vi "批次管理.vi"() -> ()   [LabVIEW 2020]
uses:
  <vilib>/addons/database/Connection.llb/DB Tools Open Connec (String).vi
  <vilib>/addons/database/Connection.llb/Conn Execute.vi
  <vilib>/addons/database/Recordset.llb/Rec Fetch Recordset Data (R).vi
  <vilib>/addons/database/Recordset.llb/Rec Destroy - Connection.vi
  Global_Variable/Global.vi
  <vilib>/addons/database/NI_Database_API.lvlib
panel:
  out "产品型号":string
  out "批次信息":string[][](table)
  # "批次管理"
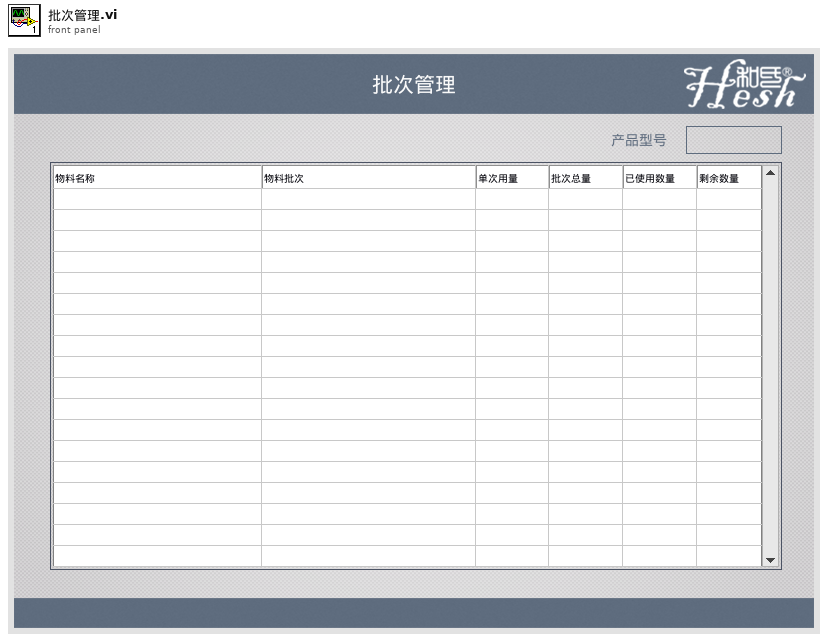
[diagram p1: front panel]
types:
  T1 = typedef "NI_Database_API.lvlib/Conn ObjectReference.ctl" = refnum<k1>
  T2 = typedef "NI_Database_API.lvlib/Rec ObjectReference.ctl" = refnum<k1>
  T3 = typedef "LVPoint32TypeDef.ctl" = cluster{"Horizontal":i32, "Vertical":i32}
  T4 = typedef "LVRowAndColumnTypeDef.ctl" = cluster{"Row":i32, "Column":i32}
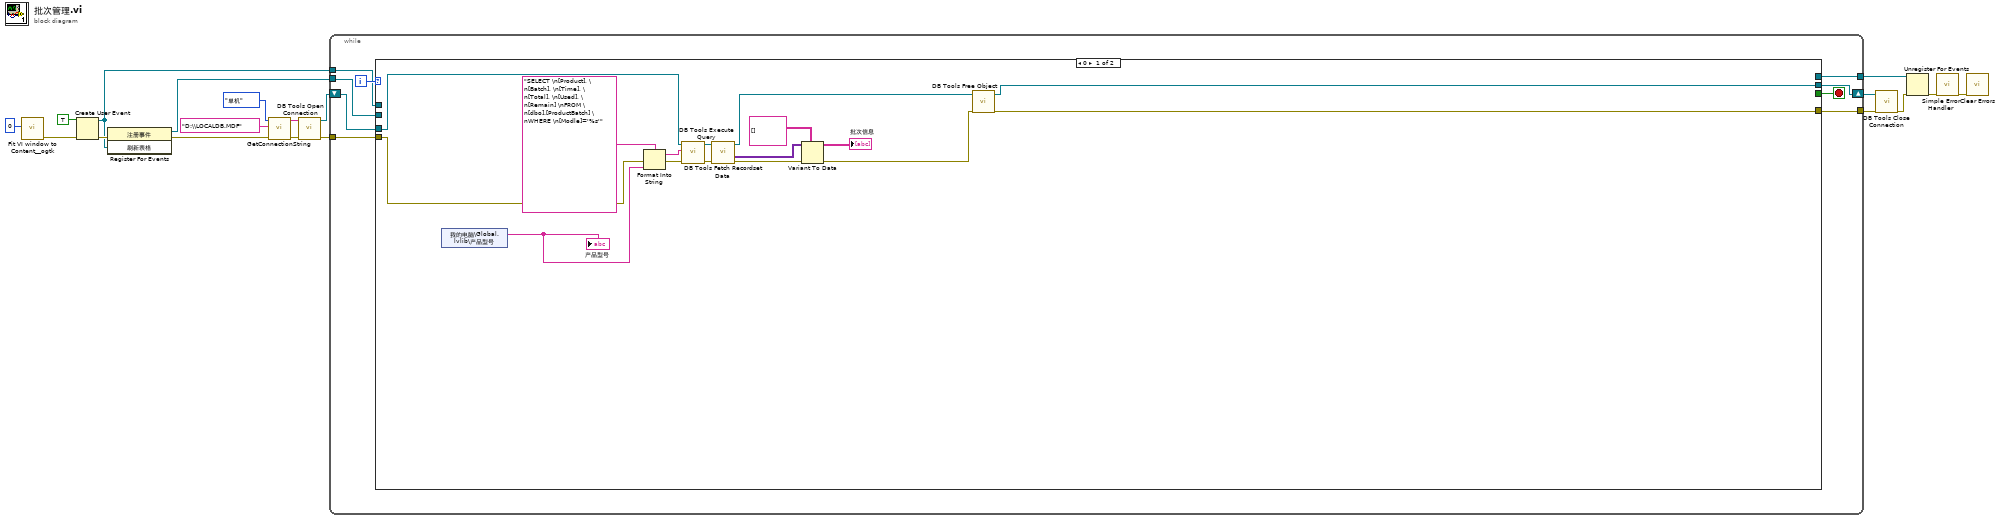
[diagram p0: block diagram]
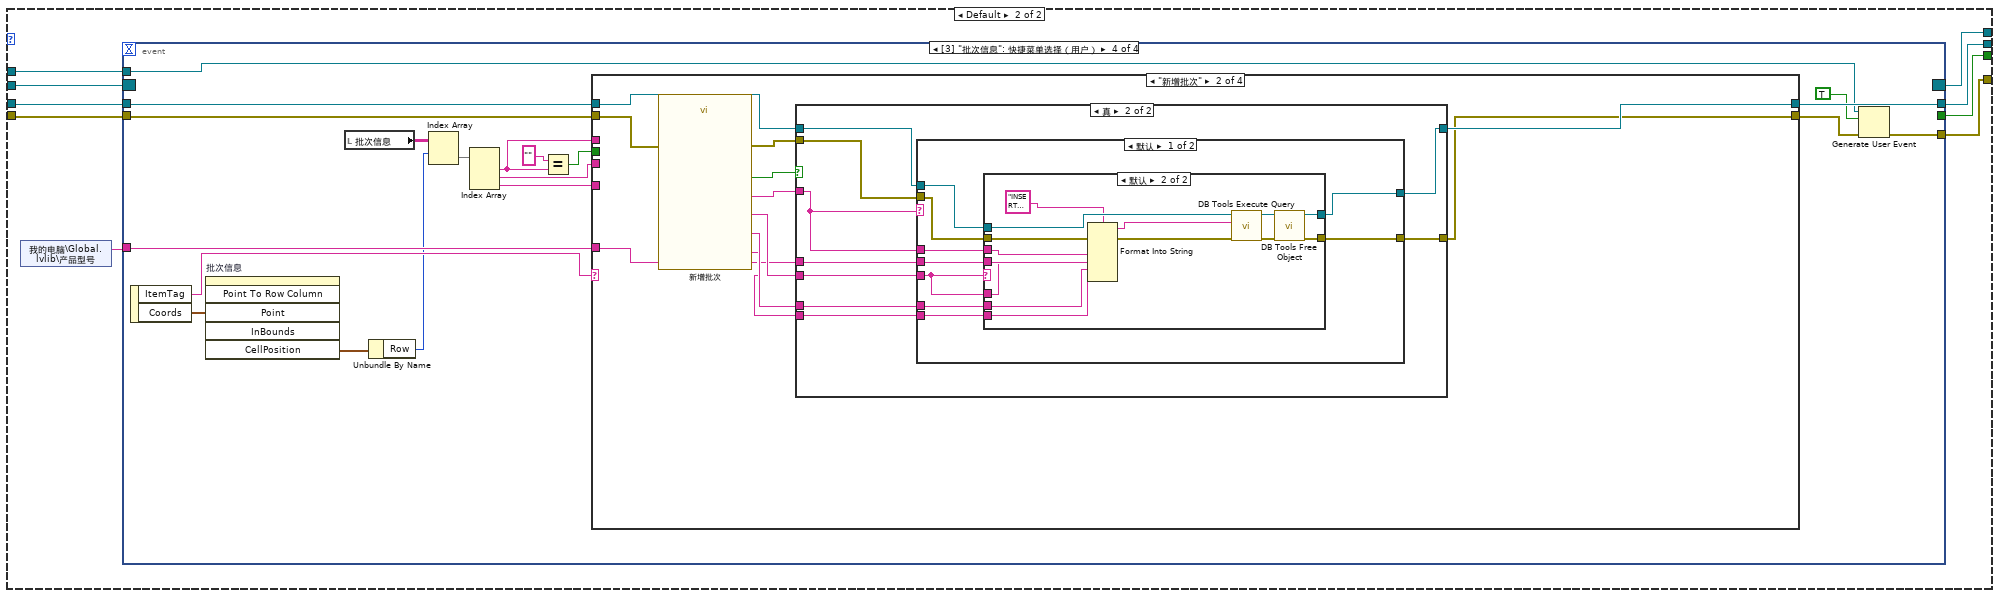
[diagram p2: hidden frame]
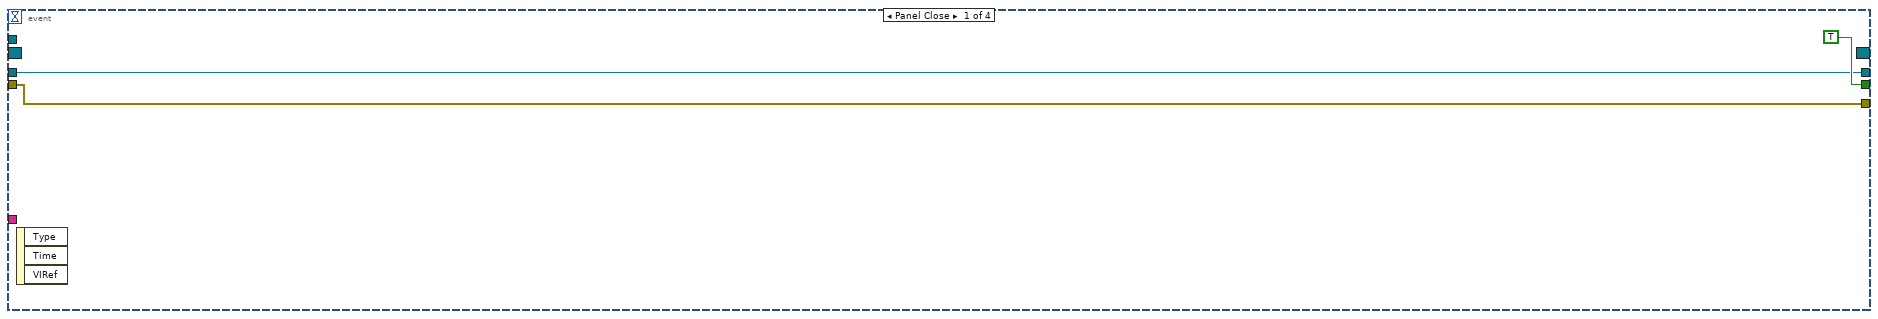
[diagram p3: hidden frame]
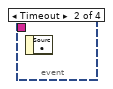
[diagram p4: hidden frame]
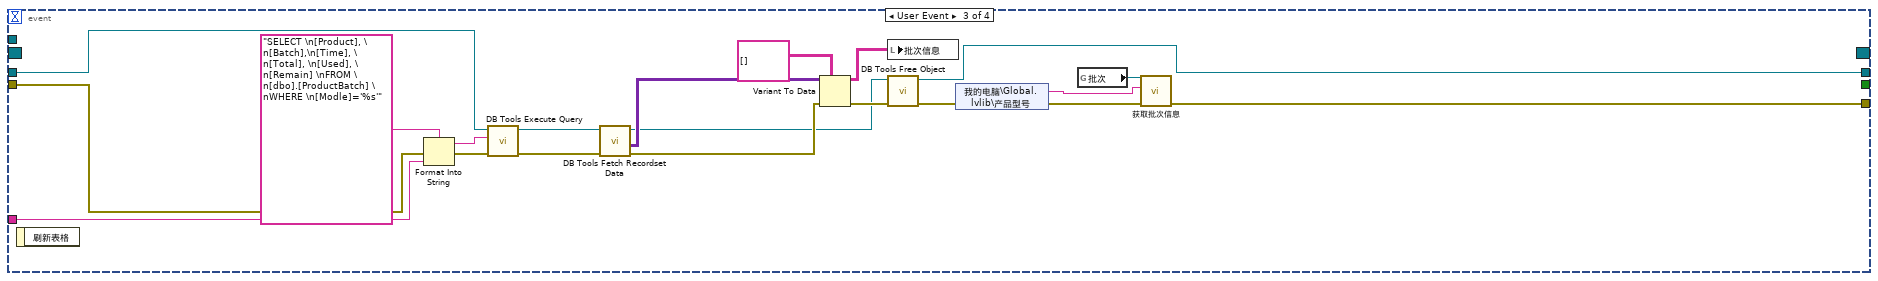
[diagram p5: hidden frame]
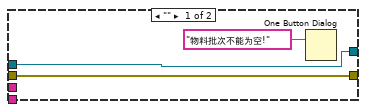
[diagram p8: hidden frame]
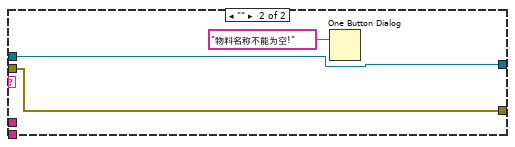
[diagram p9: hidden frame]
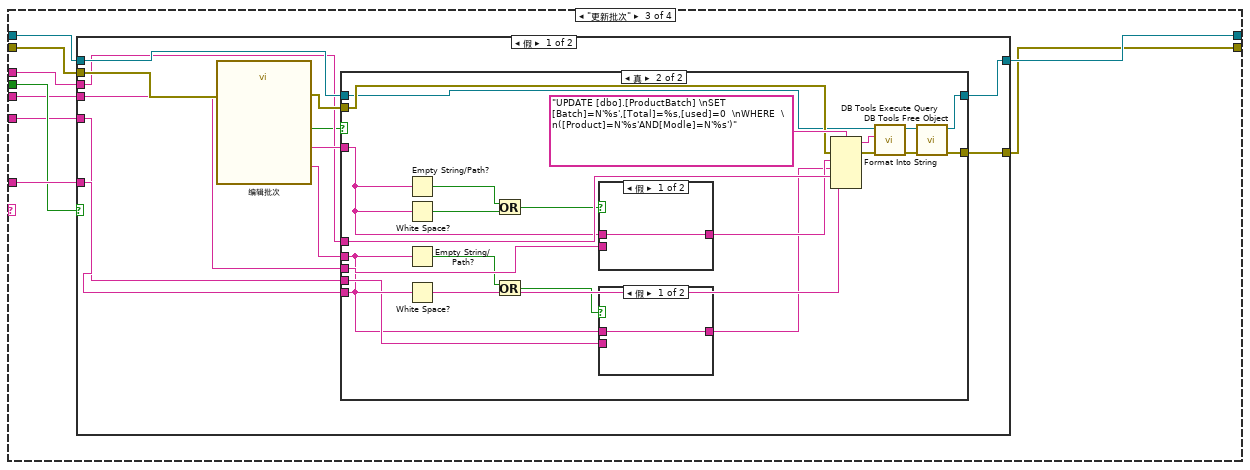
[diagram p10: hidden frame]
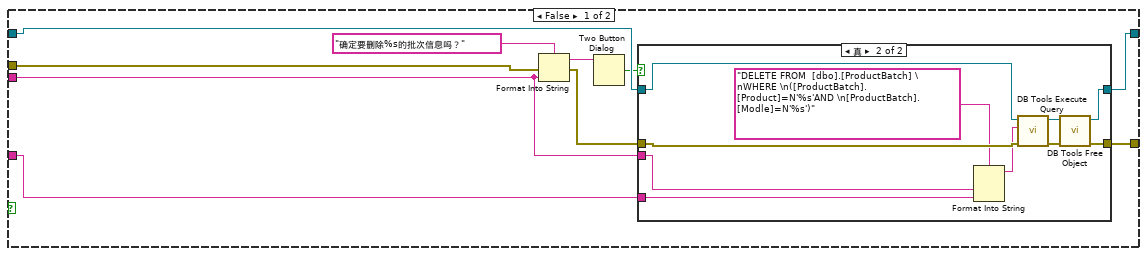
[diagram p16: hidden frame]
diagram:
  n1 = call <userlib>:"Fit VI window to Content__ogtk.vi"("border spacing (2 px)"=0) -> ("error out"=w2:errorcluster)  [unwired: 5 in, 1 out]
  n2 = Create User Event(user event datatype=TRUE ("刷新表格"), error in=w2) -> (user event=w3:refnum<user-event>, error out=w5:errorcluster)
  n3 = register-events(error in=w5, w3) -> (reference out=w11:refnum<event-registration>, error out=w7:errorcluster)  [unwired: 1 in]
  n4 = call "GetConnectionString.vi"("error in (no error)"=w7, "Database Name"="D:\\LOCALDB.MDF", "连接模式"=enum16{"单机", "联网"}."单机") -> ("error out"=w6:errorcluster, "连接字符串"=w19:string)  [unwired: 3 in]
  n5 = call-poly <vilib>:"DB Tools Open Connection.vi"("error in (no error)"=w6, "connection information"=w19) -> ("error out"=w15:errorcluster, "connection reference"=w16:T1)  [unwired: 6 in]
  n6 = while {
    tunnel: w15 -> [w26]
    tunnel: [w24] -> w13
    shift-right: [w25] -> w14
    shift-left: w16 -> [w27]
    tunnel: w11 -> [w23]
    tunnel: [w22] -> w10
    tunnel: w3 -> [w20]
    i -> [w21]
    stop <- w28 stop-if-true
    n7 = case shown="0" w21 {
      tunnel: [_ w53] -> w28
      tunnel: w27 -> [w30 w52]
      tunnel: w26 -> [w31 w51]
      tunnel: [w33 w50] -> w25
      tunnel: [w32 w49] -> w24
      tunnel: w23 -> [_ w48]
      tunnel: [_ w47] -> w22
      tunnel: w20 -> [_ w46]
      frame 0 {
        n8 = shared-variable "我的电脑\\Global.lvlib\\产品型号"() -> (w29:string)  [unwired: 1 in, 1 out]
        "产品型号" <- w29
        n9 = Format Into String(format string="SELECT \n[Product], \n[Batch], \n[Time], \n[Total], \n[Used], \n[Remain] \nFROM \n[dbo].[ProductBatch] \nWHERE \n[Modle]='%s'" ("格式字符串"), error in=w31, w29) -> (resulting string=w35:string, error out=w36:errorcluster)  [unwired: 1 in]
        n10 = call-poly <vilib>:"DB Tools Execute Query.vi"("error in (no error)"=w36, "SQL query"=w35, "connection reference"=w30) -> ("error out"=w44:errorcluster, "recordset reference"=w43:T2)  [unwired: 5 in]
        n11 = call-poly <vilib>:"DB Tools Fetch Recordset Data.vi"("error in (no error)"=w44, "recordset reference"=w43) -> ("error out"=w42:errorcluster, "recordset data"=w41:variant[][], "recordset reference out"=w38:T2)  [unwired: 3 in]
        n12 = Variant To Data(error in=w42, type=string[][] [], Variant=w41) -> (data=→"批次信息":string[][], error out=w39:errorcluster)
        n13 = call-poly <vilib>:"DB Tools Free Object.vi"("error in (no error)"=w39, "recordset reference"=w38) -> ("error out"=w32:errorcluster, "connection reference"=w33:T1)  [unwired: 8 in]
      }
      frame Default {
        n14 = shared-variable "我的电脑\\Global.lvlib\\产品型号"() -> (w45:string)  [unwired: 1 in, 1 out]
        n15 = event shown="[3] \"批次信息\": 快捷菜单选择（用户）" {
          selector: w48 -> [_ _ _ _]
          dyn-events: [_ _ _ _] -> w47
          timeout: _ -> [_ _ _ _]
          tunnel: [TRUE _ _ _] -> w53
          tunnel: w52 -> [w55 _ w66 w94]
          tunnel: w51 -> [w54 _ w64 w93]
          tunnel: [w55 _ w63 w92] -> w50
          tunnel: [w54 _ w58 w83] -> w49
          tunnel: w45 -> [_ _ w65 w91]
          tunnel: w46 -> [_ _ _ w86]
          event Panel Close {
            n16 = event-data() -> ()  [unwired: 1 in, 3 out]
          }
          event Timeout {
            n17 = event-data() -> ()  [unwired: 1 in, 1 out]
          }
          event User Event {
            n18 = event-data() -> ()  [unwired: 1 in, 1 out]
            n19 = Format Into String(format string="SELECT \n[Product], \n[Batch],\n[Time], \n[Total], \n[Used], \n[Remain] \nFROM \n[dbo].[ProductBatch] \nWHERE \n[Modle]='%s'" ("格式字符串"), error in=w64, w65) -> (resulting string=w67:string, error out=w68:errorcluster)  [unwired: 1 in]
            n20 = call-poly <vilib>:"DB Tools Execute Query.vi"("error in (no error)"=w68, "SQL query"=w67, "connection reference"=w66) -> ("error out"=w76:errorcluster, "recordset reference"=w75:T2)  [unwired: 5 in]
            n21 = call-poly <vilib>:"DB Tools Fetch Recordset Data.vi"("error in (no error)"=w76, "recordset reference"=w75) -> ("error out"=w74:errorcluster, "recordset data"=w73:variant[][], "recordset reference out"=w70:T2)  [unwired: 3 in]
            n22 = Variant To Data(error in=w74, type=string[][] [], Variant=w73) -> (data=w62:string[][], error out=w71:errorcluster)
            n23 = local write "批次信息"(w62) -> ()
            n24 = call-poly <vilib>:"DB Tools Free Object.vi"("error in (no error)"=w71, "recordset reference"=w70) -> ("error out"=w60:errorcluster, "connection reference"=w63:T1)  [unwired: 8 in]
            n25 = shared-variable "我的电脑\\Global.lvlib\\产品型号"(error in=w60) -> (w61:string, error out=w59:errorcluster)
            n26 = global read "Global.vi" "批次"() -> (w57:refnum<vi>)
            n27 = call "获取批次信息.vi"("error in (no error)"=w59, "产品型号"=w61, "Tbl引用句柄"=w57) -> ("error out"=w58:errorcluster)  [unwired: 7 in, 1 out]
          }
          event "批次信息": Shortcut Menu Selection (User) {
            n28 = event-data() -> ("ItemTag"=w95:string, "Coords"=w82:T3)  [unwired: 1 in]
            n29 = invoke on="批次信息" class="Tbl (严格)" method="Point To Row Column"("Point"=w82) -> ("CellPosition"=w81:T4)  [unwired: 5 in, 5 out]
            n30 = local read "批次信息"() -> (w88:string[][])
            n31 = Unbundle By Name(w81) -> ("Row"=w89:i32)
            n32 = Index Array(array=w88, index (row)=w89) -> (element=w80:string[])  [unwired: 1 in]
            n33 = Index Array(array=w80) -> (element #1=w79:string, element #2=w78:string, element #3=w77:string)  [unwired: 3 in]
            n34 = Equal?(x="" ("元素"), y=w79) -> (x = y?=w87:bool)
            n35 = case shown="\"新增批次\"" w95 {
              tunnel: w94 -> [w96 w108 w156 w207]
              tunnel: w93 -> [w97 w105 w155 w206]
              tunnel: [w97 w106 w151 w202] -> w84
              tunnel: [w96 w107 w152 w203] -> w92
              tunnel: w91 -> [_ w98 w157 w204]
              tunnel: w79 -> [_ _ w153 w205]
              tunnel: w87 -> [_ _ w154 w201]
              tunnel: w78 -> [_ _ w150 _]
              tunnel: w77 -> [_ _ w149 _]
              frame Default {
              }
              frame "新增批次" {
                n36 = call "新增批次"("error in (no error)"=w105) -> ("单次使用数量"=w99:string, "批次数量"=w101:string, "物料批次"=w102:string, "物料名称"=w103:string, "确定"=w104:bool, "error out"=w100:errorcluster)  [unwired: 13 in]
                n37 = case shown="真" w104 {
                  tunnel: [w109 w119] -> w106
                  tunnel: [w110 w118] -> w107
                  tunnel: w103 -> [_ w112]
                  tunnel: w102 -> [_ w113]
                  tunnel: w101 -> [_ w117]
                  tunnel: w108 -> [w110 w116]
                  tunnel: w100 -> [w109 w115]
                  tunnel: w98 -> [_ w114]
                  tunnel: w99 -> [_ w111]
                  frame False {
                  }
                  frame True {
                    n38 = case shown="默认" w112 {
                      tunnel: [w128 w147] -> w119
                      tunnel: [w127 w148] -> w118
                      tunnel: w117 -> [w126 _]
                      tunnel: w116 -> [w125 w148]
                      tunnel: w115 -> [w124 w147]
                      tunnel: w114 -> [w123 _]
                      tunnel: w112 -> [w122 _]
                      tunnel: w113 -> [w121 _]
                      tunnel: w111 -> [w120 _]
                      frame Default {
                        n39 = case shown="默认" w121 {
                          tunnel: [w129 w141] -> w128
                          tunnel: [w130 w140] -> w127
                          tunnel: w126 -> [_ w139]
                          tunnel: w125 -> [w130 w138]
                          tunnel: w124 -> [w129 w137]
                          tunnel: w123 -> [_ w136]
                          tunnel: w122 -> [_ w135]
                          tunnel: w121 -> [_ w134]
                          tunnel: w120 -> [_ w132]
                          frame "" {
                            n40 = One Button Dialog(message="物料批次不能为空!" ("消息")) -> ()  [unwired: 1 in, 1 out]
                          }
                          frame Default {
                            n41 = Format Into String(format string="INSERT INTO \n[dbo].[ProductBatch] \n([Modle], [Product],[Batch],[Total],[Time]) \nVALUES (N'%s',N'%s', N'%s',N'%s',N'%s')" ("格式字符串"), error in=w137, w136, w135, w134, w139, w132) -> (resulting string=w145:string, error out=w142:errorcluster)  [unwired: 1 in]
                            n42 = call-poly <vilib>:"DB Tools Execute Query.vi"("error in (no error)"=w142, "SQL query"=w145, "connection reference"=w138) -> ("error out"=w144:errorcluster, "recordset reference"=w143:T2)  [unwired: 5 in]
                            n43 = call-poly <vilib>:"DB Tools Free Object.vi"("error in (no error)"=w144, "recordset reference"=w143) -> ("error out"=w141:errorcluster, "connection reference"=w140:T1)  [unwired: 8 in]
                          }
                        }
                      }
                      frame "" {
                        n44 = One Button Dialog(message="物料名称不能为空!" ("消息")) -> ()  [unwired: 1 in, 1 out]
                      }
                    }
                  }
                }
              }
              frame "更新批次" {
                n45 = case shown="假" w154 {
                  tunnel: w157 -> [w164 _]
                  tunnel: w156 -> [w168 w199]
                  tunnel: w155 -> [w167 w200]
                  tunnel: w153 -> [w165 _]
                  tunnel: [w163 w199] -> w152
                  tunnel: [w162 w200] -> w151
                  tunnel: w150 -> [w160 _]
                  tunnel: w149 -> [w159 _]
                  frame False {
                    n46 = call "编辑批次"("error in (no error)"=w167) -> ("批次数量"=w158:string, "物料批次"=w166:string, "确定"=w161:bool, "error out"=w169:errorcluster)  [unwired: 15 in]
                    n47 = case shown="真" w161 {
                      tunnel: w168 -> [w171 w186]
                      tunnel: w169 -> [w170 w189]
                      tunnel: w158 -> [_ w173]
                      tunnel: [w171 w188] -> w163
                      tunnel: [w170 w187] -> w162
                      tunnel: w166 -> [_ w179]
                      tunnel: w165 -> [_ w185]
                      tunnel: w164 -> [_ w184]
                      tunnel: w160 -> [_ w182]
                      tunnel: w159 -> [_ w181]
                      frame False {
                      }
                      frame True {
                        n48 = Empty String/Path?(string/path=w179) -> (empty?=w178:bool)
                        n49 = White Space?(1:w179) -> (0:w177:bool)
                        n50 = Empty String/Path?(string/path=w173) -> (empty?=w175:bool)
                        n51 = White Space?(1:w173) -> (0:w174:bool)
                        n52 = Or(x=w178, y=w177) -> (x .or. y?=w176:bool)
                        n53 = Or(x=w175, y=w174) -> (x .or. y?=w172:bool)
                        n54 = case shown="假" w176 {
                          tunnel: w179 -> [w197 _]
                          tunnel: [w197 w198] -> w183
                          tunnel: w182 -> [_ w198]
                          frame False {
                          }
                          frame True {
                          }
                        }
                        n55 = case shown="假" w172 {
                          tunnel: w173 -> [w195 _]
                          tunnel: [w195 w196] -> w180
                          tunnel: w181 -> [_ w196]
                          frame False {
                          }
                          frame True {
                          }
                        }
                        n56 = Format Into String(format string="UPDATE [dbo].[ProductBatch] \nSET [Batch]=N'%s',[Total]=%s,[used]=0  \nWHERE  \n([Product]=N'%s'AND[Modle]=N'%s')" ("格式字符串"), error in=w189, w183, w180, w185, w184) -> (resulting string=w193:string, error out=w190:errorcluster)  [unwired: 1 in]
                        n57 = call-poly <vilib>:"DB Tools Execute Query.vi"("error in (no error)"=w190, "SQL query"=w193, "connection reference"=w186) -> ("error out"=w192:errorcluster, "recordset reference"=w191:T2)  [unwired: 5 in]
                        n58 = call-poly <vilib>:"DB Tools Free Object.vi"("error in (no error)"=w192, "recordset reference"=w191) -> ("error out"=w187:errorcluster, "connection reference"=w188:T1)  [unwired: 8 in]
                      }
                    }
                  }
                  frame True {
                  }
                }
              }
              frame "删除批次" {
                n59 = case shown="真" w201 {
                  tunnel: w205 -> [w209 _]
                  tunnel: w206 -> [w216 w230]
                  tunnel: w207 -> [w214 w231]
                  tunnel: [w212 w231] -> w203
                  tunnel: [w211 w230] -> w202
                  tunnel: w204 -> [w208 _]
                  frame False {
                    n60 = Format Into String(format string="确定要删除%s的批次信息吗？" ("格式字符串"), error in=w216, w209) -> (resulting string=w215:string, error out=w213:errorcluster)  [unwired: 1 in]
                    n61 = Two Button Dialog(message=w215) -> (T button?=w210:bool)  [unwired: 2 in]
                    n62 = case shown="真" w210 {
                      tunnel: w214 -> [w219 w229]
                      tunnel: w213 -> [w218 w228]
                      tunnel: [w219 w225] -> w212
                      tunnel: [w218 w224] -> w211
                      tunnel: w209 -> [_ w222]
                      tunnel: w208 -> [_ w220]
                      frame False {
                      }
                      frame True {
                        n63 = Format Into String(format string="DELETE FROM  [dbo].[ProductBatch] \nWHERE \n([ProductBatch].[Product]=N'%s'AND \n[ProductBatch].[Modle]=N'%s')" ("格式字符串"), w222, w220) -> (resulting string=w221:string)  [unwired: 2 in, 1 out]
                        n64 = call-poly <vilib>:"DB Tools Execute Query.vi"("error in (no error)"=w228, "SQL query"=w221, "connection reference"=w229) -> ("error out"=w227:errorcluster, "recordset reference"=w226:T2)  [unwired: 5 in]
                        n65 = call-poly <vilib>:"DB Tools Free Object.vi"("error in (no error)"=w227, "recordset reference"=w226) -> ("error out"=w224:errorcluster, "connection reference"=w225:T1)  [unwired: 8 in]
                      }
                    }
                  }
                  frame True {
                  }
                }
              }
            }
            n66 = Generate User Event(user event=w86, event data cluster=TRUE ("事件数据"), error in=w84) -> (error out=w83:errorcluster)  [unwired: 1 in, 1 out]
          }
        }
      }
    }
  }
  n67 = call <vilib>:"DB Tools Close Connection.vi"("error in (no error)"=w13, "connection reference"=w14) -> ("error out"=w9:errorcluster)  [unwired: 5 in]
  n68 = Unregister For Events(event registration refnum=w10, error in=w9) -> (error out=w8:errorcluster)
  n69 = call <vilib>:"Simple Error Handler.vi"("error in (no error)"=w8) -> ("error out"=w12:errorcluster)  [unwired: 4 in, 4 out]
  n70 = call <vilib>:"Clear Errors.vi"("error in (no error)"=w12) -> ()  [unwired: 5 in, 2 out]
